vi "AFG3352X.set GaussLL.vi"(2 "error in (no error)":errorcluster, 4 "length [us]":dbl=0.02 format="%^#.3e", 5 "VISA in":refnum<visa-resource-name>="GPIB0::8::INSTR") -> (0 "error out":errorcluster, 1 "VISA out":refnum<visa-resource-name>)   [LabVIEW 2014, in "AFG3352X.lvlib"]
doc: "Low-level part of the Gaussian programming procedure. Included in this class since\nI did not want it to be confused with the VERY low-level stuff in the LabVIEW instr.lib.\n\nHistory: JULY-2004, Stefan Schwarz"
uses:
  AFG3352X.lvlib
  CSinstr.lib/Agilent 3352X Series/Agilent 3352X Series.lvlib
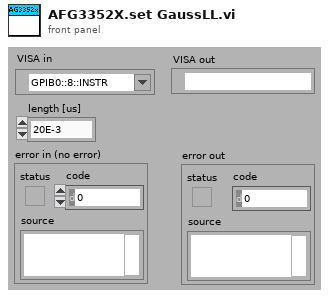
[diagram p1: front panel]
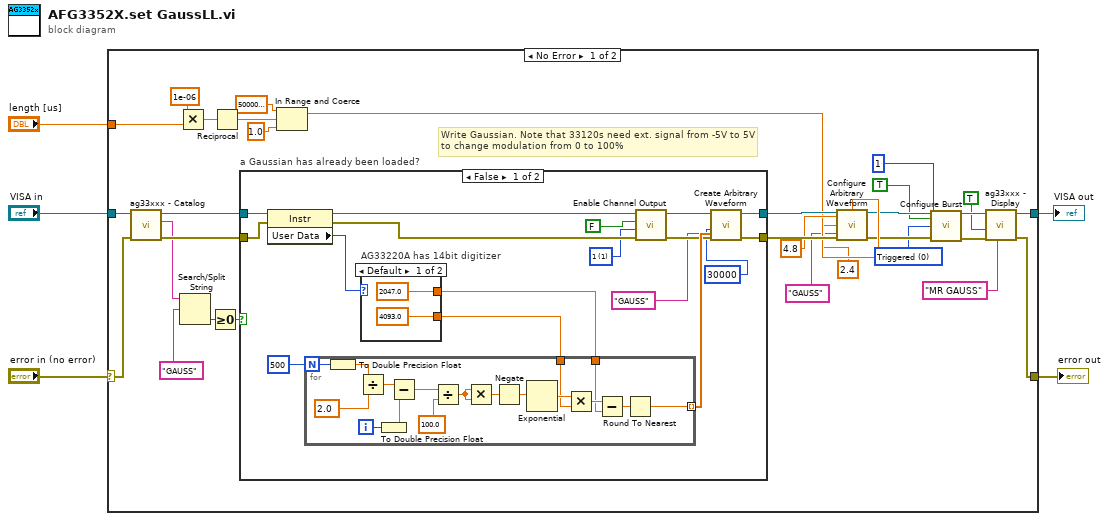
[diagram p0: block diagram]
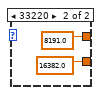
[diagram p2: hidden frame]
diagram:
  n1 = case shown="No Error" "error in (no error)" {
    selector: "error in (no error)" -> [w18 w77]
    tunnel: "length [us]" -> [w36 _]
    tunnel: "VISA in" -> [w19 w78]
    tunnel: [w8 w77] -> w3
    tunnel: [w10 w78] -> w2
    frame No Error {
      w23 = u16 0 items=["Triggered", "Gated"] ("Burst Modulation Mode (0: Triggered)")
      # "Write Gaussian. Note that 33120s need ext. signal from -5V to 5V\nto change modulation from 0 to 100%"
      n2 = call "ag33xxx - Catalog.vi"("error in (no error)"=w18, "VISA session"=w19) -> ("error out"=w16:errorcluster, "Catalog"=w13:string, "dup VISA session"=w17:refnum<visa-resource-name>)  [unwired: 7 in]
      n3 = Multiply(x=1e-06 ("upper limit"), y=w36) -> (x*y=w27:dbl)
      n4 = Search/Split String(string=w13, search string/char (-)="GAUSS") -> (offset of match=w15:i32)  [unwired: 1 in, 2 out]
      n5 = Greater Or Equal To 0?(x=w15) -> (x >= 0?=w14:bool)
      n6 = Reciprocal(x=w27) -> (1/x=w35:dbl)
      n7 = case "a Gaussian has already been loaded?" shown="False" w14 {
        tunnel: [w48 w76] -> w31
        tunnel: [w47 w75] -> w30
        tunnel: w17 -> [w45 w76]
        tunnel: w16 -> [w44 w75]
        frame False {
          w38 = u16 1 items=["1"=1, "2"=2] ("Channel (1: 1)")
          n8 = property class="Instr"(reference=w45, error in=w44) -> (reference out=w42:refnum<visa-resource-name>, error out=w43:errorcluster, "User Data"=w41:u32)
          n9 = case "AG33220A has 14bit digitizer" shown="Default" w41 {
            tunnel: [4093.0 ("y") 16382.0 ("y")] -> w40
            tunnel: [2047.0 ("y") 8191.0 ("y")] -> w39
            frame Default {
            }
            frame 33220 {
            }
          }
          n10 = for {
            N: 500 -> [w73]
            tunnel: [w60] -> w52 mode=indexing
            tunnel: w40 -> [w59]
            tunnel: w39 -> [w58]
            i -> [w74]
            n11 = To Double Precision Float(number=w73) -> (double precision float=w71:dbl)
            n12 = Divide(x=w71, y=2.0) -> (x/y=w70:dbl)
            n13 = To Double Precision Float(number=w74) -> (double precision float=w69:dbl)
            n14 = Subtract(x=w70, y=w69) -> (x-y=w68:dbl)
            n15 = Divide(x=w68, y=100.0) -> (x/y=w67:dbl)
            n16 = Multiply(x=w67, y=w67) -> (x*y=w66:dbl)
            n17 = Negate(x=w66) -> (-x=w65:dbl)
            n18 = Exponential(1:w65) -> (0:w64:dbl)
            n19 = Multiply(x=w64, y=w59) -> (x*y=w63:dbl)
            n20 = Subtract(x=w63, y=w58) -> (x-y=w62:dbl)
            n21 = Round To Nearest(number=w62) -> (nearest integer value=w60:dbl)
          }
          n22 = call "Enable Channel Output.vi"("error in (no error)"=w43, "Channel (1: 1)"=w38, "Enable Output (T: Enable)"=FALSE, "VISA resource name"=w42) -> ("error out"=w50:errorcluster, "VISA resource name out"=w51:refnum<visa-resource-name>)  [unwired: 6 in]
          n23 = call "Create Arbitrary Waveform.vi"("Arbitrary Waveform Data"=w52, "Arbitrary Waveform Name (ARB1)"="GAUSS", "error in (no error)"=w50, "Timeout (10000 ms)"=u32 30000 ("Timeout (10000)"), "VISA resource name"=w51) -> ("error out"=w47:errorcluster, "VISA resource name out"=w48:refnum<visa-resource-name>)  [unwired: 5 in]
        }
        frame True {
        }
      }
      n24 = In Range and Coerce(upper limit=5000000.0, x=w35, lower limit=1.0) -> (coerced(x)=w28:dbl)  [unwired: 1 out]
      n25 = call "Configure Arbitrary Waveform.vi"("VISA resource name"=w31, "Amplitude (0.1 Vpp)"=w28, "Sample Rate (40000 Sa/s)"=2.4 ("Offset (0.00 V)"), "Offset (0 V)"=4.8 ("Gain (1.0)"), "error in (no error)"=w30, "Arbitrary Waveform (ARB1)"="GAUSS") -> ("VISA resource name out"=w25:refnum<visa-resource-name>, "error out"=w24:errorcluster)  [unwired: 8 in]
      n26 = call "Configure Burst.vi"("VISA resource name"=w25, "Enable Burst (T: Enable)"=TRUE ("Enable Burst Modulation (True)"), "Channel (1: 1)"=1 ("Burst Count (1)"), "Burst Mode (0: Triggered)"=w23, "error in (no error)"=w24) -> ("VISA resource name out"=w11:refnum<visa-resource-name>, "error out"=w9:errorcluster)  [unwired: 9 in]
      n27 = call "ag33xxx - Display.vi"("Display Text"="MR GAUSS", "error in (no error)"=w9, "Text (F: off)"=TRUE, "VISA session"=w11) -> ("error out"=w8:errorcluster, "dup VISA session"=w10:refnum<visa-resource-name>)  [unwired: 6 in]
    }
    frame Error {
    }
  }
  "error out" <- w3
  "VISA out" <- w2
